vi "converter_Craig_to_Jonas.vi"(6 "theta5Craig":dbl, 7 "theta4Craig":dbl, 8 "theta6Craig":dbl, 9 "theta3Craig":dbl, 10 "theta2Craig":dbl, 11 "theta1Craig":dbl) -> (0 "theta5Jonas":dbl, 1 "theta4Jonas":dbl, 2 "theta3Jonas":dbl, 3 "theta2Jonas":dbl, 4 "theta6Jonas":dbl, 5 "theta1Jonas":dbl)   [LabVIEW 2017]
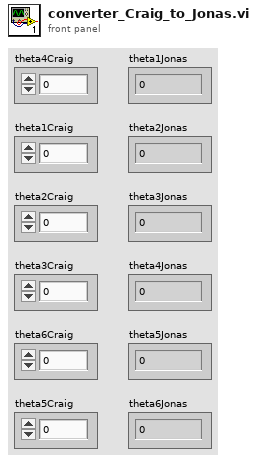
[diagram p1: front panel]
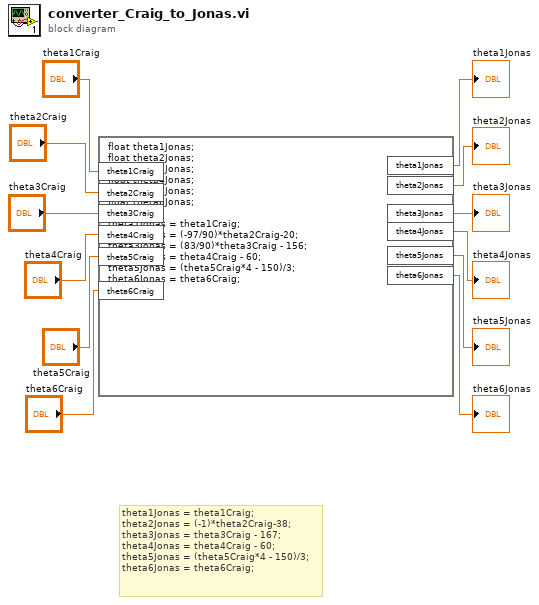
[diagram p0: block diagram]
diagram:
  # "theta1Jonas = theta1Craig;\ntheta2Jonas = (-1)*theta2Craig-38;\ntheta3Jonas = theta3Craig - 167;\ntheta4Jonas = theta4Craig - 60;\ntheta5Jonas = (theta5Craig*4 - 150)/3;\ntheta6Jonas = theta6Craig;"
  n1 = formula code="float theta1Jonas;\nfloat theta2Jonas;\nfloat theta3Jonas;\nfloat theta4Jonas;\nfloat theta5Jonas;\nfloat theta6Jonas;\n\ntheta1Jonas = theta1Craig;\ntheta2Jonas = (-97/90)*theta2Craig-20;\ntheta3Jonas = (83/90)*theta3Craig - 156;\ntheta4Jonas = theta4Craig - 60;\ntheta5Jonas = (theta5Craig*4 - 150)/3;\ntheta6Jonas = theta6Craig;"("theta1Craig"="theta1Craig", "theta3Craig"="theta3Craig", "theta4Craig"="theta4Craig", "theta5Craig"="theta5Craig", "theta6Craig"="theta6Craig", "theta2Craig"="theta2Craig") -> ("theta1Jonas"=→"theta1Jonas":dbl, "theta2Jonas"=→"theta2Jonas":dbl, "theta3Jonas"=→"theta3Jonas":dbl, "theta4Jonas"=→"theta4Jonas":dbl, "theta5Jonas"=→"theta5Jonas":dbl, "theta6Jonas"=→"theta6Jonas":dbl)
